vi "read_attributes.vi"(8 "error in (no error)":errorcluster, 11 "Perceptron in":refnum<class "Perceptron.lvclass">) -> (0 "error out":errorcluster, 2 "attributes":T1, 3 "Perceptron out":refnum<class "Perceptron.lvclass">)   [LabVIEW 2020, in "Perceptron.lvclass"]
uses:
  Perceptron.lvclass
  Controls/perceptron_attributes.ctl
  Perceptron.lvclass/Perceptron.ctl
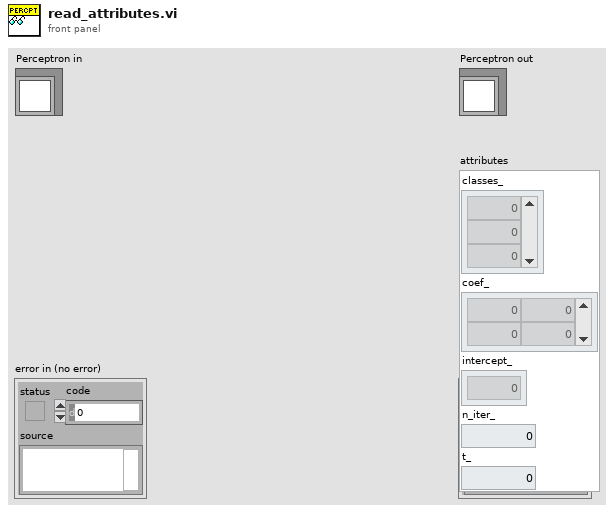
[diagram p1: front panel]
types:
  T1 = typedef "perceptron_attributes.ctl" = cluster{"classes_":dbl[], "coef_":dbl[][], "intercept_":dbl[], "n_iter_":dbl, "t_":dbl}
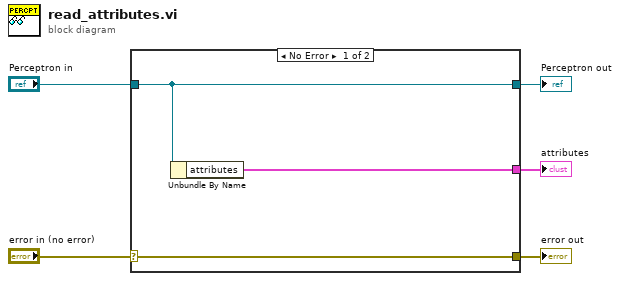
[diagram p0: block diagram]
diagram:
  n1 = case shown="No Error" "error in (no error)" {
    selector: "error in (no error)" -> [w8 w9]
    tunnel: [w8 w9] -> w4
    tunnel: [w7 w10] -> w2
    tunnel: "Perceptron in" -> [w7 w10]
    tunnel: [w6 _] -> w1
    frame No Error {
      n2 = Unbundle By Name(w7) -> ("attributes"=w6:T1)
    }
    frame Error {
    }
  }
  "error out" <- w4
  "Perceptron out" <- w2
  "attributes" <- w1
